vi "index_two_axes.vi"(8 "x_index":i32, 11 "graph_data":cluster{"array type (2D Dbl)":dbl[], dbl[]}[](array[cluster])) -> (2 "Y2":dbl, 3 "Y1":dbl, 5 "X":dbl)   [LabVIEW 2025]
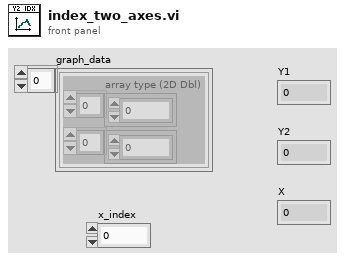
[diagram p1: front panel]
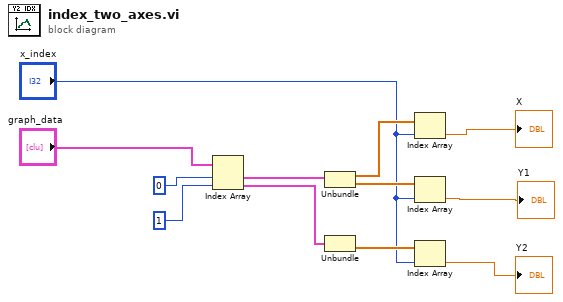
[diagram p0: block diagram]
diagram:
  n1 = Index Array(array="graph_data", index #1=0 ("index"), index #2=1 ("index")) -> (element #1=w6:cluster{"array type (2D Dbl)":dbl[], dbl[]}, element #2=w3:cluster{"array type (2D Dbl)":dbl[], dbl[]})
  n2 = Unbundle(w6) -> ("array type (2D Dbl)"=w8:dbl[], w5:dbl[])
  n3 = Unbundle(w3) -> (w4:dbl[])  [unwired: 1 out]
  n4 = Index Array(array=w8, index="x_index") -> (element=→"X":dbl)
  n5 = Index Array(array=w5, index="x_index") -> (element=→"Y1":dbl)
  n6 = Index Array(array=w4, index="x_index") -> (element=→"Y2":dbl)
